vi "openMeas.vi"(8 "error in":errorcluster, 11 "FPGA VI (in)":T1) -> (0 "error out":errorcluster, 1 "Nsamples":u32, 3 "FPGA VI (out)":T1)   [LabVIEW 2021]
uses:
  <vilib>/rvi/interface/nirviReadWriteControl/nirviReadWriteControl.xnode
  <vilib>/rvi/interface/nirviMethod/nirviMethod.xnode
  acdc-PV-emulators/FPGA Bitfiles/FPGA.ctl
  <vilib>/rvi/errors/niLvFpgaMergeErrorWithErrorCode.vi
panel:
  in  "dF [Hz]":fxp<+,36,5>
  in  "window samples":i32=3000
  in  "N ch":u32=6
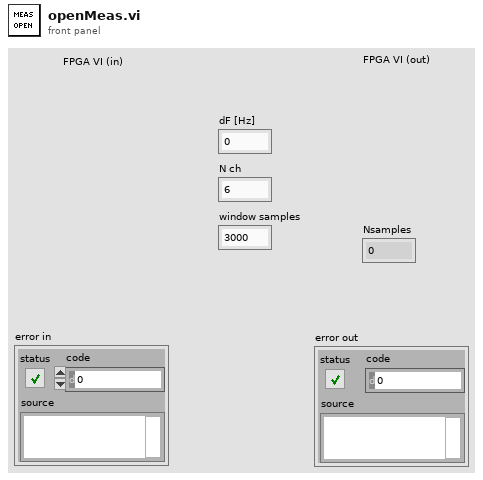
[diagram p1: front panel]
types:
  T1 = typedef "FPGA.ctl" = refnum<k20>
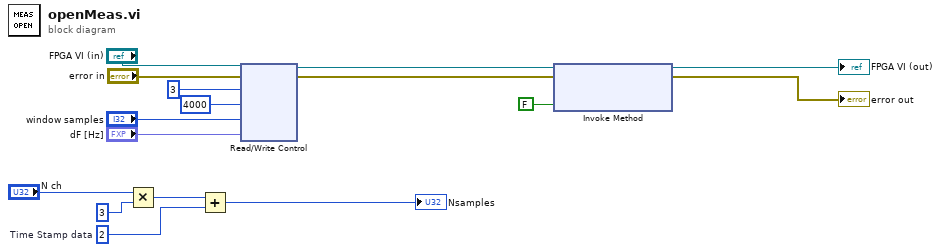
[diagram p0: block diagram]
diagram:
  w16 = u32 2  # Time Stamp data
  n1 = Multiply(x="N ch", y=u32 3) -> (x*y=w15:u32)
  n2 = Add(x=w15, y=w16) -> (x+y=→"Nsamples":u32)
  n3 = xnode "Read/Write Control"("FPGA VI Reference In"="FPGA VI (in)", "error in"="error in", "iMAX"=u16 3, "CB Size"=u16 4000, "N"="window samples", "dF [Hz]"="dF [Hz]") -> ("FPGA VI Reference Out"=w6:T1, "error out"=w5:errorcluster)
  n4 = xnode "Invoke Method"("FPGA VI Reference In"=w6, "error in"=w5, "Wait Until Done (F)"=FALSE) -> ("FPGA VI Reference Out"=→"FPGA VI (out)":T1, "error out"=→"error out":errorcluster)
